vi "top_format_plots.vi"(8 "error in":errorcluster, 9 "Front panel refs":T3, 10 "Dynamic data":T1, 11 "Input parameters":T2={"Measurement type"=enum."Debug", "Sensor type"=enum."IFX_8in_256ch", "Identifier"="test.txt", "Open after execution?"=FALSE, "Plot after execution?"=FALSE, "Display channel"=0, "Voltage Delay (s)"=0.5, "Switch Delay (s)"=0.01, "VISA resource name source"="", "VISA resource name DMM"="", "VISA resource name LCR"="", "Compliance  Level (A)"=1e-05, "Voltage Limit (V)"=1000.0, "Data storage location"="", "Scan voltages"="", "Use source as DMM?"=FALSE, "LCR signal frequenzy (Hz)"=10000.0, "DMM device"=enum."Keithley2450", "Sampling number"=1, "Use env. sensors on"=enum."Sensirion sht1x/7x", "Switchboard Handle"=0, "Use Switchboard"=FALSE, "LCR signal voltage (V)"=10000.0, "Repeat"=1, "Scan voltages IV"="", "Scan voltages CV"="", "Hex pad numbers?"=FALSE, "Set measurement type"=enum."Debug", "Custom pad scan"="", "IV voltage Delay (s)"=0.5, "CV voltage Delay (s)"=0.5, "Needle measurement?"=FALSE, "Comments"="test.txt", "LCR signal frequenzy (kHz)"=10.0, "Compliance  Level (uA)"=10.0, "Open Correction Array"=array2304x3[6912 elements], "Current set voltage"=0.0, "Last set voltage"=0.0, "Current channel"=0, "Last OpenCorrection index"=-1, "Total curr/vltg every x steps"=10, "Current channel iteration"=0, "No CV corrections"=FALSE, "Mapfile"="", "Corrfile"="", "IV voltage file"=path "", "CV voltage file"=path "", "IV Switch Delay (s)"=0.01, "CV Switch Delay (s)"=0.01, "Invert polarity"=FALSE, "Set debug dirs"=FALSE, "Is n on p"=FALSE} {"CV Switch Delay (s)" format="%#_13g"; "IV Switch Delay (s)" format="%#_13g"; "Last set voltage" format="%#_13g"; "Current set voltage" format="%#_13g"; "CV voltage Delay (s)" format="%#_13g"; "IV voltage Delay (s)" format="%#_13g"; "Voltage Limit (V)" format="%#_13g"; "Voltage Delay (s)" format="%#_13g"; "Switch Delay (s)" format="%#_13g"}) -> (0 "error out":errorcluster, 1 "Front panel refs out":T3, 2 "Dynamic data out":T1, 3 "Input parameters out":T2={"Measurement type"=enum."Debug", "Sensor type"=enum."IFX_8in_256ch", "Identifier"="test.txt", "Open after execution?"=FALSE, "Plot after execution?"=FALSE, "Display channel"=0, "Voltage Delay (s)"=0.5, "Switch Delay (s)"=0.01, "VISA resource name source"="", "VISA resource name DMM"="", "VISA resource name LCR"="", "Compliance  Level (A)"=1e-05, "Voltage Limit (V)"=1000.0, "Data storage location"="", "Scan voltages"="", "Use source as DMM?"=FALSE, "LCR signal frequenzy (Hz)"=10000.0, "DMM device"=enum."Keithley2450", "Sampling number"=1, "Use env. sensors on"=enum."Sensirion sht1x/7x", "Switchboard Handle"=0, "Use Switchboard"=FALSE, "LCR signal voltage (V)"=10000.0, "Repeat"=1, "Scan voltages IV"="", "Scan voltages CV"="", "Hex pad numbers?"=FALSE, "Set measurement type"=enum."Debug", "Custom pad scan"="", "IV voltage Delay (s)"=0.5, "CV voltage Delay (s)"=0.5, "Needle measurement?"=FALSE, "Comments"="test.txt", "LCR signal frequenzy (kHz)"=10.0, "Compliance  Level (uA)"=10.0, "Open Correction Array"=array2304x3[6912 elements], "Current set voltage"=0.0, "Last set voltage"=0.0, "Current channel"=0, "Last OpenCorrection index"=-1, "Total curr/vltg every x steps"=10, "Current channel iteration"=0, "No CV corrections"=FALSE, "Mapfile"="", "Corrfile"="", "IV voltage file"=path "", "CV voltage file"=path "", "IV Switch Delay (s)"=0.01, "CV Switch Delay (s)"=0.01, "Invert polarity"=FALSE, "Set debug dirs"=FALSE, "Is n on p"=FALSE} {"CV Switch Delay (s)" format="%#_13g"; "IV Switch Delay (s)" format="%#_13g"; "Last set voltage" format="%#_13g"; "Current set voltage" format="%#_13g"; "CV voltage Delay (s)" format="%#_13g"; "IV voltage Delay (s)" format="%#_13g"; "Voltage Limit (V)" format="%#_13g"; "Voltage Delay (s)" format="%#_13g"; "Switch Delay (s)" format="%#_13g"})   [LabVIEW 2016]
doc: "Formats the plots depending on user input."
uses:
  input_params.ctl
  refs_front_panel.ctl
  data_dynamic.ctl
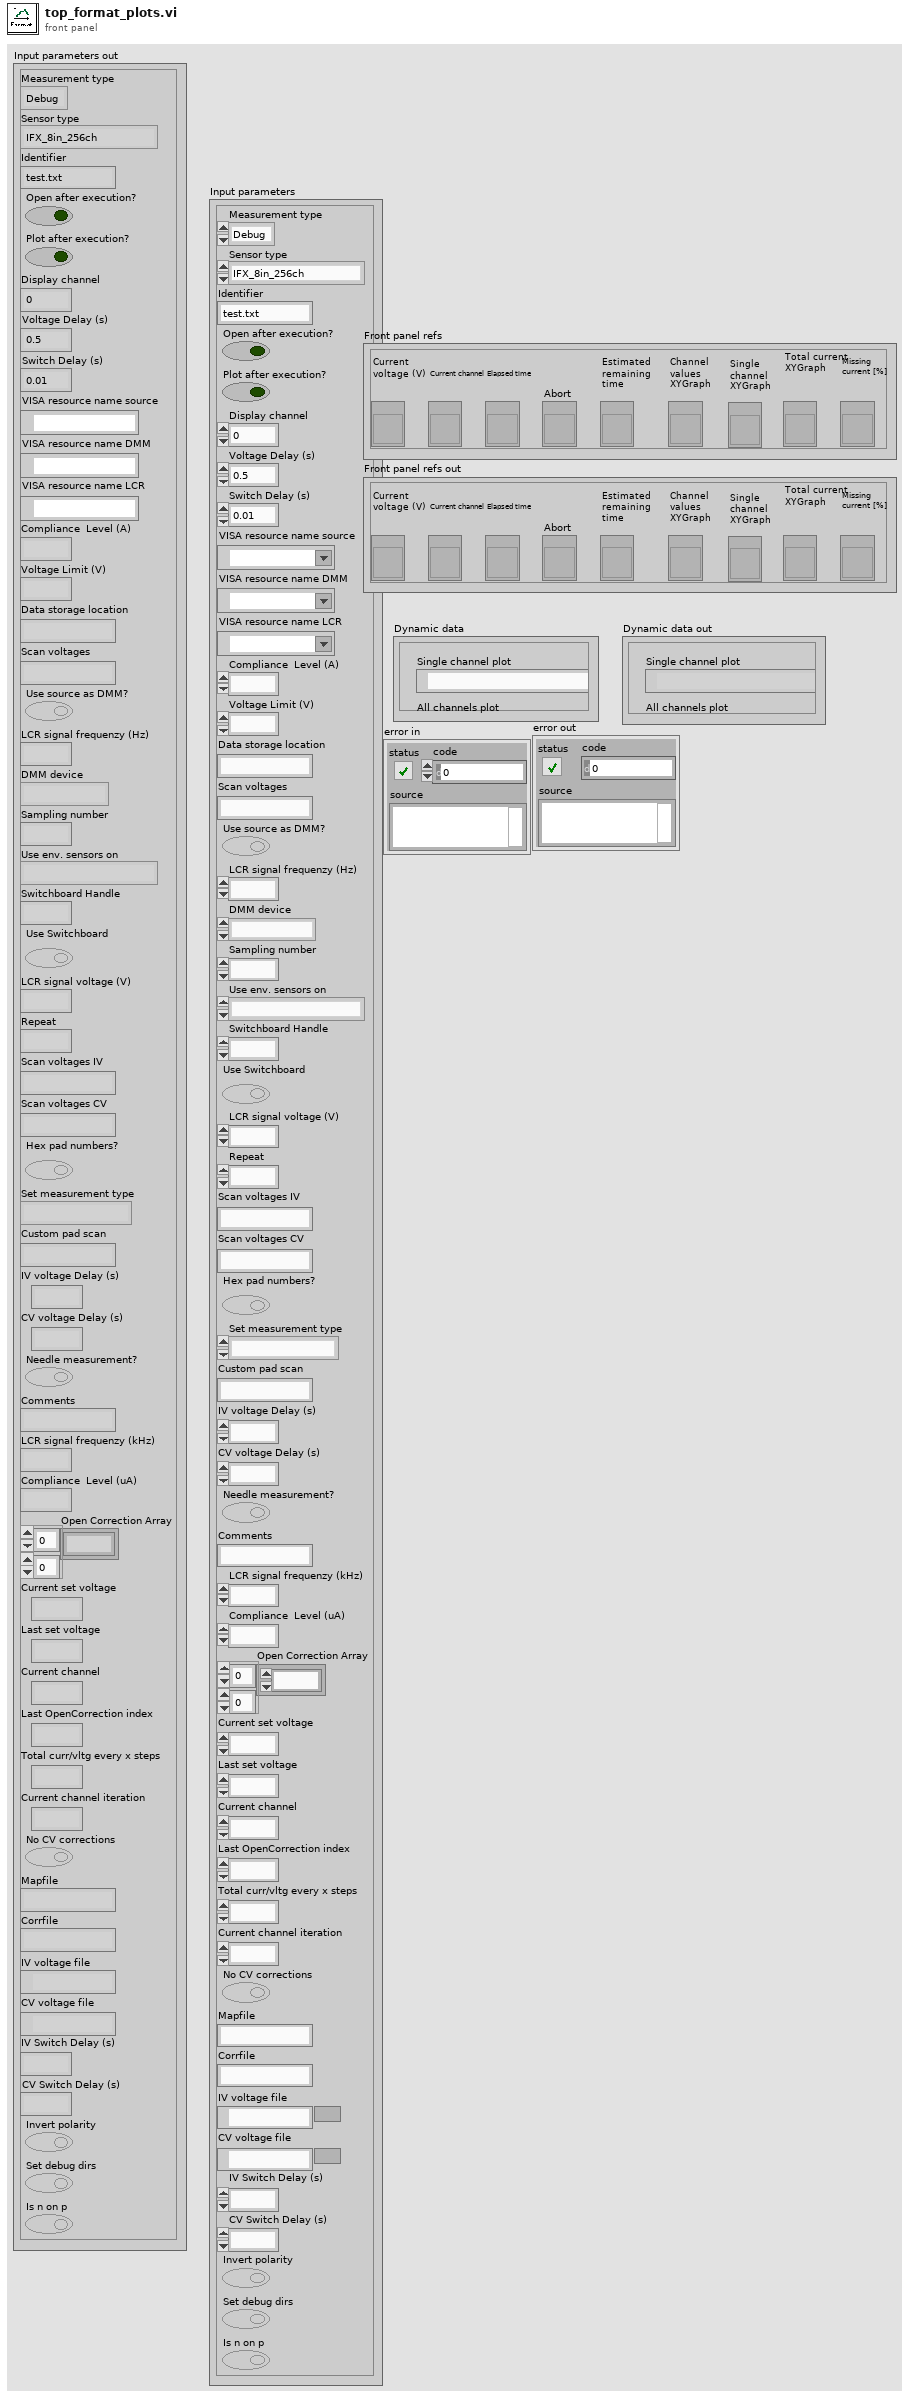
[diagram p1: front panel]
types:
  T1 = typedef "data_dynamic.ctl" = cluster{"Output file":path, "Y-label text":string, "Current set voltage":dbl, "Set voltage column":dbl[], "Pad number column":dbl[], "Data  column":dbl[], "Number of voltages":i32, "Compliance current (A)":dbl, "Geofile":string, "Peak voltage":dbl, "Hex PDF file":string, "Voltage array":dbl[], "Total current column":dbl[], "Timestamp column":dbl[], "Data name":string, "Data unit":string, "2nd data column":dbl[], "2nd data name":string, "2nd data unit":string, "3rd data column":dbl[], "4th data column":dbl[], "3rd data name":string, "3rd data unit":string, "4th data name":string, "4th data unit":string, "Actual voltage column":dbl[], "2nd Y-label text":string, "Single channel plot":path, "Temperature column":dbl[], "Humidity column":dbl[], "Channel switch array":i32[], "1st single plot name":string, "2nd single plot name":string, "All channels plot":path, "HexPlot command":string, "Custom channel array":i32[], "Data  error column":dbl[], "2nd data  error column":dbl[], "3rd data error column":dbl[], "4th data  error column":dbl[], "Total current plot":path, "5th data column":dbl[], "5th data  error column":dbl[], "6th data column":dbl[], "6th data  error column":dbl[], "5th data name":string, "5th data unit":string, "6th data name":string, "6th data unit":string, "HexPlot matrix command":string}
  T2 = typedef "input_params.ctl" = cluster{"Measurement type":enum16{"IV", "CV", "Debug", "Test_contact"}, "Sensor type":enum16{"HPK_6in_135ch", "HPK_8in_256ch", "IFX_8in_256ch", "Diode", "HPK_6in_256ch", "Full_Matrix", ""}, "Identifier":string, "Open after execution?":bool, "Plot after execution?":bool, "Display channel":i32, "Voltage Delay (s)":dbl, "Switch Delay (s)":dbl, "VISA resource name source":refnum<visa-resource-name>, "VISA resource name DMM":refnum<visa-resource-name>, "VISA resource name LCR":refnum<visa-resource-name>, "Compliance  Level (A)":dbl, "Voltage Limit (V)":dbl, "Data storage location":string, "Scan voltages":string, "Use source as DMM?":bool, "LCR signal frequenzy (Hz)":dbl, "DMM device":enum16{"Keithley2001", "Keithley2450", "Keithley2410", "Keithley6487"}, "Sampling number":i32, "Use env. sensors on":enum16{"Sensirion sht1x/7x", "Switch Matrix", "Probecard"}, "Switchboard Handle":u32, "Use Switchboard":bool, "LCR signal voltage (V)":dbl, "Repeat":i32, "Scan voltages IV":string, "Scan voltages CV":string, "Hex pad numbers?":bool, "Set measurement type":enum16{"IV", "CV", "Debug", "Test_contact", "IV+CV"}, "Custom pad scan":string, "IV voltage Delay (s)":dbl, "CV voltage Delay (s)":dbl, "Needle measurement?":bool, "Comments":string, "LCR signal frequenzy (kHz)":dbl, "Compliance  Level (uA)":dbl, "Open Correction Array":dbl[][], "Current set voltage":dbl, "Last set voltage":dbl, "Current channel":i32, "Last OpenCorrection index":i32, "Total curr/vltg every x steps":i32, "Current channel iteration":i32, "No CV corrections":bool, "Mapfile":string, "Corrfile":string, "IV voltage file":path, "CV voltage file":path, "IV Switch Delay (s)":dbl, "CV Switch Delay (s)":dbl, "Invert polarity":bool, "Set debug dirs":bool, "Is n on p":bool}
  T3 = typedef "refs_front_panel.ctl" = cluster{"Current voltage (V)":refnum<vi>, "Elapsed time":refnum<vi>, "Current channel":refnum<vi>, "Abort":refnum<vi>, "Estimated remaining time":refnum<vi>, "Channel values XYGraph":refnum<vi>, "Single channel XYGraph":refnum<vi>, "Total current XYGraph":refnum<vi>, "Missing\ncurrent [%]":refnum<vi>}
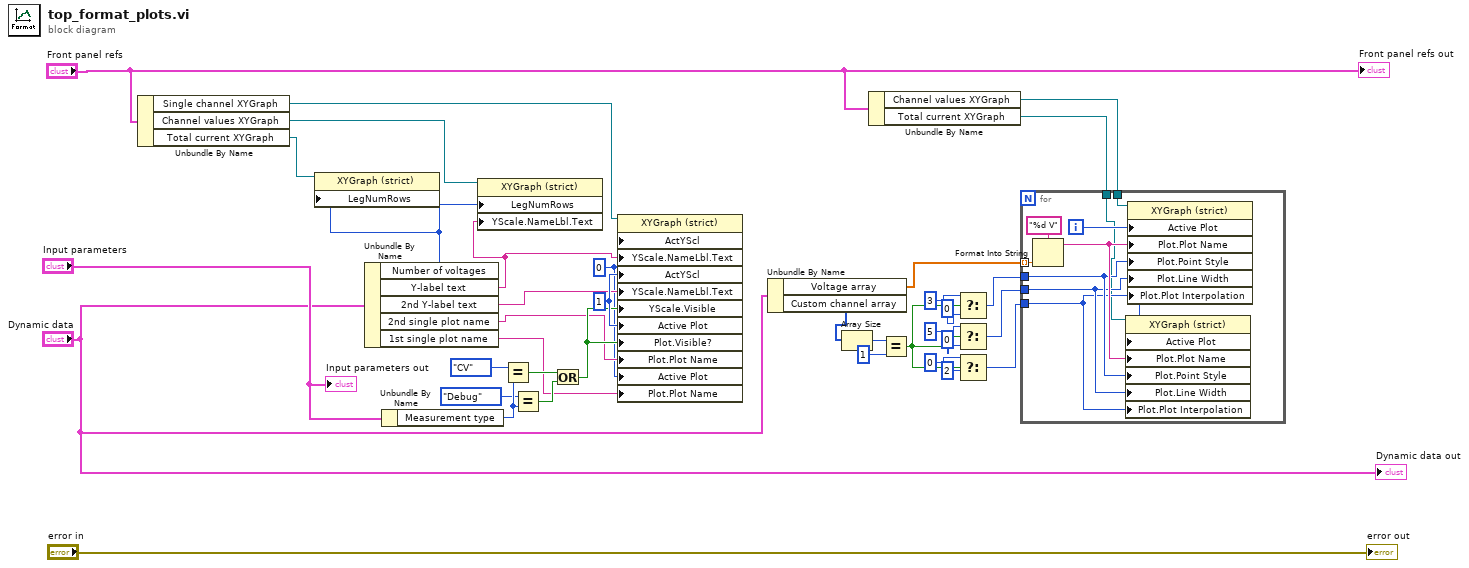
[diagram p0: block diagram]
diagram:
  w22 = 1 ("Active Y Scale")
  w17 = 0 ("Active Y Scale")
  n1 = Unbundle By Name("Front panel refs") -> ("Single channel XYGraph"=w7:refnum<vi>, "Channel values XYGraph"=w8:refnum<vi>, "Total current XYGraph"=w9:refnum<vi>)
  n2 = Unbundle By Name("Dynamic data") -> ("Number of voltages"=w10:i32, "Y-label text"=w23:string, "2nd Y-label text"=w21:string, "2nd single plot name"=w19:string, "1st single plot name"=w18:string)
  n3 = property on="Property Node" class="XYGraph (strict)"(reference=w9, "LegNumRows"=w10) -> ()  [unwired: 1 in, 2 out]
  n4 = Unbundle By Name("Input parameters") -> ("Measurement type"=w25:enum16{"IV", "CV", "Debug", "Test_contact"})
  n5 = property on="Property Node" class="XYGraph (strict)"(reference=w8, "LegNumRows"=w10, "YScale.NameLbl.Text"=w23) -> ()  [unwired: 1 in, 2 out]
  n6 = Equal?(x=enum16{"IV", "CV", "Debug", "Test_contact"}."CV", y=w25) -> (x = y?=w27:bool)
  n7 = Equal?(x=enum16{"IV", "CV", "Debug", "Test_contact"}."Debug", y=w25) -> (x = y?=w26:bool)
  n8 = Or(x=w27, y=w26) -> (x .or. y?=w20:bool)
  n9 = property on="Property Node" class="XYGraph (strict)"(reference=w7, "ActYScl"=w17, "YScale.NameLbl.Text"=w23, "ActYScl"=w22, "YScale.NameLbl.Text"=w21, "YScale.Visible"=w20, "Active Plot"=w22, "Plot.Visible?"=w20, "Plot.Plot Name"=w19, "Active Plot"=w17, "Plot.Plot Name"=w18) -> ()  [unwired: 1 in, 2 out]
  n10 = Unbundle By Name("Dynamic data") -> ("Voltage array"=w24:dbl[], "Custom channel array"=w11:i32[])
  n11 = Array Size(array=w11) -> (size(s)=w14:i32)
  n12 = Unbundle By Name("Front panel refs") -> ("Channel values XYGraph"=w5:refnum<vi>, "Total current XYGraph"=w4:refnum<vi>)
  n13 = Equal?(x=w14, y=1) -> (x = y?=w12:bool)
  n14 = Select(t=u8 3 ("Plot.Point Style"), s=w12, f=u8 0 ("Plot.Point Style")) -> (s? t:f=w28:u8)
  n15 = Select(t=u8 5 ("Plot.Point Style"), s=w12, f=u8 0 ("Plot.Point Style")) -> (s? t:f=w29:u8)
  n16 = Select(t=u8 0 ("Plot.Point Style"), s=w12, f=u8 2 ("Plot.Point Style")) -> (s? t:f=w30:u8)
  n17 = for {
    tunnel: w30 -> [w40]
    tunnel: w29 -> [w41]
    tunnel: w28 -> [w42]
    tunnel: w24 -> [w44] mode=indexing
    tunnel: w5 -> [w38]
    tunnel: w4 -> [w37]
    i -> [w39]
    n18 = Format Into String(format string="%d V", w44) -> (resulting string=w43:string)  [unwired: 2 in, 1 out]
    n19 = property on="Property Node" class="XYGraph (strict)"(reference=w37, "Active Plot"=w39, "Plot.Plot Name"=w43, "Plot.Point Style"=w42, "Plot.Line Width"=w41, "Plot.Plot Interpolation"=w40) -> ()  [unwired: 1 in, 2 out]
    n20 = property on="Property Node" class="XYGraph (strict)"(reference=w38, "Active Plot"=w39, "Plot.Plot Name"=w43, "Plot.Point Style"=w42, "Plot.Line Width"=w41, "Plot.Plot Interpolation"=w40) -> ()  [unwired: 1 in, 2 out]
  }
  "Front panel refs out" <- "Front panel refs"
  "Input parameters out" <- "Input parameters"
  "Dynamic data out" <- "Dynamic data"
  "error out" <- "error in"
